vi "Delete Project Temporary Files Wrapper.vi"(8 "error in (no error)":errorcluster, 11 "LabVIEW Build Script in":refnum<class "LabVIEW Build Script.lvclass">) -> (0 "error out":errorcluster)   [LabVIEW 2021, in "LabVIEW Build Script.lvclass"]
uses:
  LabVIEW Build Script.lvclass
  LabVIEW Build Script.lvclass/LabVIEW Build Script.ctl
  Build Script Common/Build Script Common.lvlib
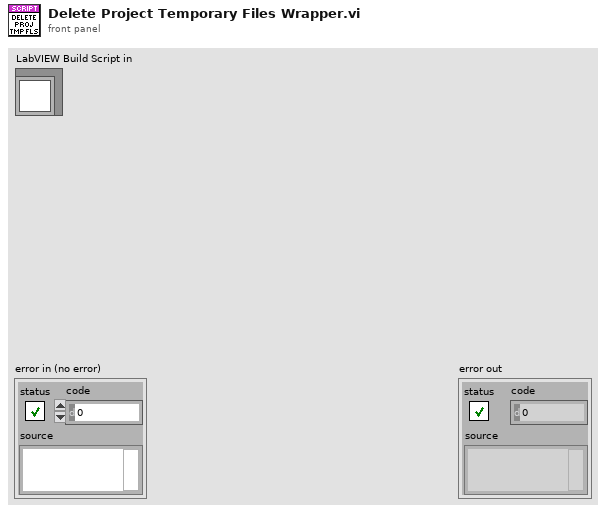
[diagram p1: front panel]
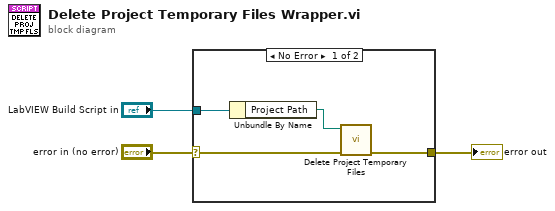
[diagram p0: block diagram]
diagram:
  n1 = case shown="No Error" "error in (no error)" {
    selector: "error in (no error)" -> [w5 w8]
    tunnel: [w4 w8] -> w2
    tunnel: "LabVIEW Build Script in" -> [w7 _]
    frame No Error {
      n2 = Unbundle By Name(w7) -> ("Project Path"=w6:path)
      n3 = call "Delete Project Temporary Files.vi"("error in (no error)"=w5, "Project Path"=w6) -> ("error out"=w4:errorcluster)  [unwired: 9 in]
    }
    frame Error {
    }
  }
  "error out" <- w2
